vi "Demo_Data Re-arrange.vi"(8 "error In":errorcluster, 11 "Data In":T2) -> (0 "error Out":errorcluster, 3 "Data Out":T1)   [LabVIEW 2017]
uses:
  <vilib>/addons/database/Auxilliary.llb/DB Tools Format Datetime String (Time Stamp).vi
  <vilib>/addons/database/NI_Database_API.lvlib
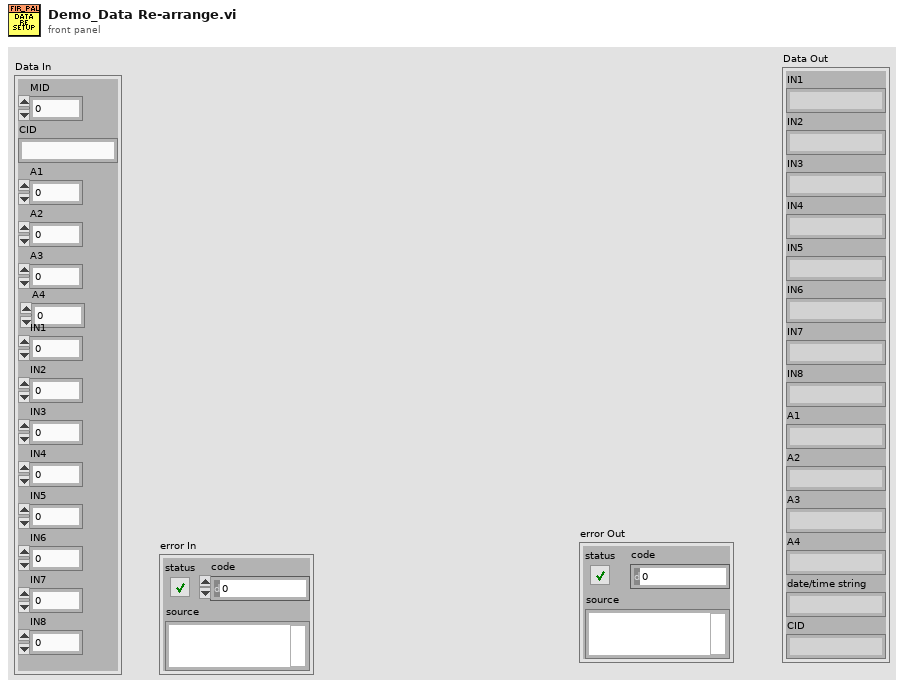
[diagram p1: front panel]
types:
  T1 = cluster{"IN1":string, "IN2":string, "IN3":string, "IN4":string, "IN5":string, "IN6":string, "IN7":string, "IN8":string, "A1":string, "A2":string, "A3":string, "A4":string, "date/time string":string, "CID":string}
  T2 = cluster{"MID":dbl, "CID":string, "A1":dbl, "A2":dbl, "A3":dbl, "IN1":u8, "IN2":u8, "IN3":u8, "IN4":u8, "IN5":u8, "IN6":u8, "IN7":u8, "IN8":u8, "A4":dbl}
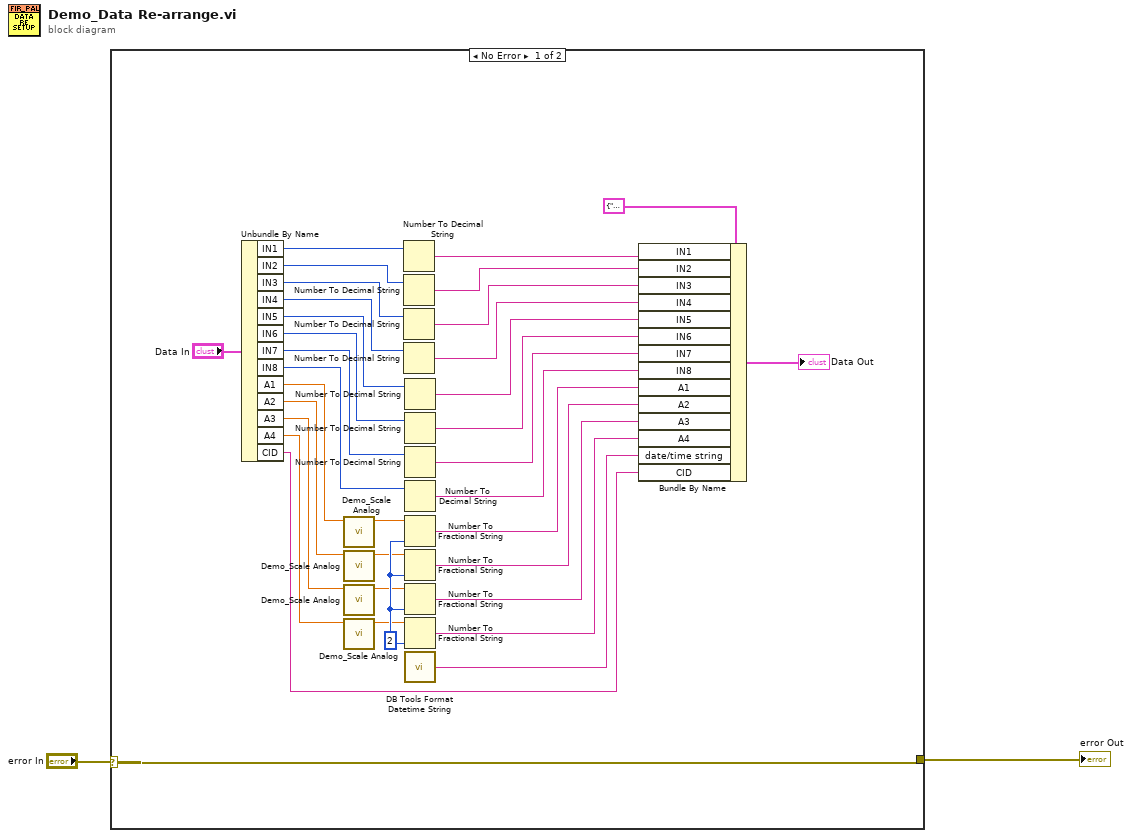
[diagram p0: block diagram]
diagram:
  n1 = case shown="No Error" "error In" {
    selector: "error In" -> [w28 w38]
    tunnel: [w28 w38] -> w1
    frame No Error {
      w18 = i16 2 ("precision (6)")
      n2 = Unbundle By Name("Data In") -> ("IN1"=w27:u8, "IN2"=w26:u8, "IN3"=w25:u8, "IN4"=w24:u8, "IN5"=w23:u8, "IN6"=w22:u8, "IN7"=w21:u8, "IN8"=w20:u8, "A1"=w6:dbl, "A2"=w5:dbl, "A3"=w4:dbl, "A4"=w3:dbl, "CID"=w13:string)
      n3 = call "Demo_Scale Analog.vi"("Analog IN"=w6) -> ("Calibration OUT"=w10:dbl)  [unwired: 10 in]
      n4 = call "Demo_Scale Analog.vi"("Analog IN"=w5) -> ("Calibration OUT"=w9:dbl)  [unwired: 10 in]
      n5 = call "Demo_Scale Analog.vi"("Analog IN"=w4) -> ("Calibration OUT"=w8:dbl)  [unwired: 10 in]
      n6 = call "Demo_Scale Analog.vi"("Analog IN"=w3) -> ("Calibration OUT"=w7:dbl)  [unwired: 10 in]
      n7 = Number To Decimal String(number=w27) -> (decimal integer string=w29:string)  [unwired: 1 in]
      n8 = Number To Decimal String(number=w26) -> (decimal integer string=w30:string)  [unwired: 1 in]
      n9 = Number To Decimal String(number=w25) -> (decimal integer string=w31:string)  [unwired: 1 in]
      n10 = Number To Decimal String(number=w24) -> (decimal integer string=w32:string)  [unwired: 1 in]
      n11 = Number To Decimal String(number=w23) -> (decimal integer string=w34:string)  [unwired: 1 in]
      n12 = Number To Decimal String(number=w22) -> (decimal integer string=w35:string)  [unwired: 1 in]
      n13 = Number To Decimal String(number=w21) -> (decimal integer string=w36:string)  [unwired: 1 in]
      n14 = Number To Decimal String(number=w20) -> (decimal integer string=w37:string)  [unwired: 1 in]
      n15 = Number To Fractional String(number=w10, precision (6)=w18) -> (F-format string=w17:string)  [unwired: 2 in]
      n16 = Number To Fractional String(number=w9, precision (6)=w18) -> (F-format string=w16:string)  [unwired: 2 in]
      n17 = Number To Fractional String(number=w8, precision (6)=w18) -> (F-format string=w15:string)  [unwired: 2 in]
      n18 = Number To Fractional String(number=w7, precision (6)=w18) -> (F-format string=w14:string)  [unwired: 2 in]
      n19 = call-poly <vilib>:"DB Tools Format Datetime String.vi"() -> ("date/time string"=w19:string)  [unwired: 1 in]
      n20 = Bundle By Name(cluster=T1 {"IN1"="", "IN2"="", "IN3"="", "IN4"="", "IN5"="", "IN6"="", "IN7"="", "IN8"="", "A1"="", "A2"="", "A3"="", "A4"="", "date/time string"="", "CID"=""}, "IN1"=w29, "IN2"=w30, "IN3"=w31, "IN4"=w32, "IN5"=w34, "IN6"=w35, "IN7"=w36, "IN8"=w37, "A1"=w17, "A2"=w16, "A3"=w15, "A4"=w14, "date/time string"=w19, "CID"=w13) -> (→"Data Out":T1)
    }
    frame Error {
    }
  }
  "error Out" <- w1
